vi "diffraction pattern v1.0.vi"() -> ()   [LabVIEW 2019]
panel:
  in  "Exit":bool
  in  "Run":bool
  out "Help":string="1. before run, set the paramaters on the left of the screen.\n2. flux (magnetic field) is in unit of flux quanta.\n3. Phaserange is in the unit of Pi, the CPR will be build up according to phase range of [-Phaserange/2,Phaserang/2], and such CPR will be  a periodic function with Phaserange as period. Enter integer number  of multiple times of 4 is preferred.\n4. Use the step setting tab to set resolution of the calculation, you can set how many points is used to define the width of the Josephson junction, how many points to represent the Phaserange\n5. Then you can choose which type of the CPR is used.\n6. Depending on the choose of the CPR, you may want to set the strength of the MBS, \"a\" parameter, the width of the gaussian function used, and the pattern of parity of MBS. Parity pattern has to have same number of elements for positive and negative range.\nEnter the parity 1 or -1 for positive and negative phase +-Pi, +-3Pi, +-5Pi etc.. in to the two arrays.\n7. You can use the index control to read the array elements, then enter the value, you can also delete an element of array by right click, the number of array elements is not limited.\n8. You can change the x,y range, zoom, create cursor etc. to help analyse the plot. Right click to save the data into excel.\n\nEnjoy!\nGuang Yue\n\n\n"
  in  "parity for negative phase":i32[](array[numeric])=[1, -1, -1, 1]
  in  "Strenth of MBS":dbl=0.5
  in  "parity for positive phase":i32[](array[numeric])=[1, -1, 1, 1]
  in  "Gaussian width":dbl=0.2
  in  "Tab Control":enum32{"Range", "Steps setting"}(tab)=enum."Steps setting"
  in  "flux start":dbl=-6.0
  in  "flux end":dbl=6.0
  in  "flux step":dbl=0.05
  in  "phaserange in Pi":i32=16
  in  "Geometry":i32=501
  in  "Phase steps":i32=501
  in  "CPR Type":T1(ring)=enum."Local MBS different parity"
  out "Total time s":dbl=20.42792349999945
  in  "stop loop":bool
  out "Diffraction pattern plot":cluster{cluster{dbl, "icn":dbl}[]}[](graph)=[{[{-6.0, "icn"=0.015201191288397739}, {-5.95, "icn"=0.01969262363818792}, {-5.9, "icn"=0.02816050403543407}, {-5.85, "icn"=0.03640577475812925}, {-5.8, "icn"=0.0442230884309362}, {-5.75, "icn"=0.05141409458211041}, {-5.7, "icn"=0.05779064505501809}, {-5.65, "icn"=0.06315912943628797}, {-5.6, "icn"=0.06721764065757277}, {-5.55, "icn"=0.06967553141250711}, {-5.5, "icn"=0.07013136060103732}, {-5.45, "icn"=0.06873370042025707}, {-5.4, "icn"=0.06529768198713366}, {-5.35, "icn"=0.06131135129764386}, {-5.3, "icn"=0.05712967537493866}, {-5.25, "icn"=0.05172563118780871}, {-5.2, "icn"=0.04512609278717199}, {-5.15, "icn"=0.03746288339324653}, {-5.1, "icn"=0.028906304270791668}, {-5.05, "icn"=0.019652598502870128}, {-5.0, "icn"=0.009919054928091782}, {-4.95, "icn"=0.01606737269953319}, {-4.9, "icn"=0.02621287150537696}, {-4.85, "icn"=0.036114718326525894}, {-4.8, "icn"=0.04552470847214177}, {-4.75, "icn"=0.05420143525490187}, {-4.7, "icn"=0.06191253761599668}, {-4.65, "icn"=0.06840325841911396}, {-4.6, "icn"=0.07337440089453802}, {-4.55, "icn"=0.07633960072265523}, {-4.5, "icn"=0.07694003757440993}, {-4.45, "icn"=0.07511288466626331}, {-4.4, "icn"=0.07094489106760657}, {-4.35, "icn"=0.06609689508373423}, {-4.3, "icn"=0.060931348029548554}, {-4.25, "icn"=0.05424909028223394}, {-4.2, "icn"=0.046059052595585265}, {-4.15, "icn"=0.03651979778138212}, {-4.1, "icn"=0.025834109202385443}, {-4.05, "icn"=0.014238092057178582}, {-4.0, "icn"=0.0019958503876323364}, {-3.9499999999999997, "icn"=0.010606220441872604}, {-3.9, "icn"=0.02326579038953691}, {-3.85, "icn"=0.03567147774513779}, {-3.8, "icn"=0.04751011276467433}, {-3.75, "icn"=0.05847437639350753}, {-3.6999999999999997, "icn"=0.06827384015050382}, {-3.65, "icn"=0.07669046186501231}, {-3.5999999999999996, "icn"=0.08435009902148928}, {-3.55, "icn"=0.09245040955594146}, {-3.5, "icn"=0.09818699818823985}, {-3.4499999999999997, "icn"=0.100890355120277}, {-3.4, "icn"=0.1004922625302631}, {-3.3499999999999996, "icn"=0.09706827829921433}, {-3.3, "icn"=0.09102426894947412}, {-3.25, "icn"=0.0827017030407996}, {-3.1999999999999997, "icn"=0.07233356294110323}, {-3.15, "icn"=0.06012975230451682}, {-3.0999999999999996, "icn"=0.046337743528162244}, {-3.05, "icn"=0.031250380479597245}, {-3.0, "icn"=0.015201191288398029}, {-2.9499999999999997, "icn"=0.02830046911314805}, {-2.9, "icn"=0.045606743446444754}, {-2.8499999999999996, "icn"=0.06271657669902271}, {-2.8, "icn"=0.07920905924934873}, {-2.75, "icn"=0.09466404490553904}, {-2.6999999999999997, "icn"=0.10868019873668189}, {-2.65, "icn"=0.12096184118712497}, {-2.5999999999999996, "icn"=0.13242531670888072}, {-2.55, "icn"=0.14449040955831893}, {-2.5, "icn"=0.15333287915372715}, {-2.4499999999999997, "icn"=0.15827148991751971}, {-2.4, "icn"=0.15853115847796279}, {-2.3499999999999996, "icn"=0.15489608459229445}, {-2.3, "icn"=0.1473321409279046}, {-2.25, "icn"=0.1364457543320676}, {-2.1999999999999997, "icn"=0.1224918472564987}, {-2.15, "icn"=0.10570069114472812}, {-2.0999999999999996, "icn"=0.0863674182534983}, {-2.05, "icn"=0.06485938540260895}, {-2.0, "icn"=0.04161187308992893}, {-1.9500000000000002, "icn"=0.06414199436705846}, {-1.8999999999999995, "icn"=0.09146312929875294}, {-1.8499999999999996, "icn"=0.11899756797085131}, {-1.7999999999999998, "icn"=0.1461262821875672}, {-1.75, "icn"=0.1722082272120952}, {-1.7000000000000002, "icn"=0.19658288396804854}, {-1.6499999999999995, "icn"=0.2184833976597425}, {-1.5999999999999996, "icn"=0.23659141533150718}, {-1.5499999999999998, "icn"=0.2498989153464729}, {-1.5, "icn"=0.2563220452314678}, {-1.4500000000000002, "icn"=0.2562842985268351}, {-1.3999999999999995, "icn"=0.24891519362535802}, {-1.3499999999999996, "icn"=0.2402432283340347}, {-1.2999999999999998, "icn"=0.22935682894260606}, {-1.25, "icn"=0.21279197567562266}, {-1.1999999999999993, "icn"=0.19021652655761598}, {-1.1499999999999995, "icn"=0.161624706006115}, {-1.0999999999999996, "icn"=0.12714683881730285}, {-1.0499999999999998, "icn"=0.0870252060665998}, {-1.0, "icn"=0.041611873089929}, {-0.9499999999999993, "icn"=0.09203583246104262}, {-0.8999999999999995, "icn"=0.15118411815627344}, {-0.8499999999999996, "icn"=0.21448578493954668}, {-0.7999999999999998, "icn"=0.28129040253853854}, {-0.75, "icn"=0.3508881885566983}, {-0.6999999999999993, "icn"=0.4224868106416624}, {-0.6499999999999995, "icn"=0.4948894711833411}, {-0.5999999999999996, "icn"=0.5661544315062148}, {-0.5499999999999998, "icn"=0.6323635438059886}, {-0.5, "icn"=0.6900329469436456}, {-0.4499999999999993, "icn"=0.7362703178024443}, {-0.39999999999999947, "icn"=0.7698525588790502}, {-0.34999999999999964, "icn"=0.810752483754053}, {-0.2999999999999998, "icn"=0.8578720391382381}, {-0.25, "icn"=0.8998638401870045}, {-0.1999999999999993, "icn"=0.9351626723633593}, {-0.14999999999999947, "icn"=0.9631769325077864}, {-0.09999999999999964, "icn"=0.9834888354480831}, {-0.04999999999999982, "icn"=0.9957976963002162}, {0.0, "icn"=0.9999210442038277}, {0.05000000000000071, "icn"=0.9957976963002159}, {0.10000000000000053, "icn"=0.9834888354480825}, {0.15000000000000036, "icn"=0.9631769325077865}, {0.20000000000000018, "icn"=0.9351626723633573}, {0.25, "icn"=0.8998638401870053}, {0.3000000000000007, "icn"=0.8578720391382365}, {0.35000000000000053, "icn"=0.8107524837540525}, {0.40000000000000036, "icn"=0.7698525588790497}, {0.4500000000000002, "icn"=0.7362703178024449}, {0.5, "icn"=0.6900329469436458}, {0.5500000000000007, "icn"=0.6323635438059875}, {0.6000000000000005, "icn"=0.5661544315062141}, {0.6500000000000004, "icn"=0.49488947118334015}, {0.7000000000000002, "icn"=0.42248681064166155}, {0.75, "icn"=0.35088818855669884}, {0.8000000000000007, "icn"=0.281290402538538}, {0.8500000000000005, "icn"=0.2144857849395455}, {0.9000000000000004, "icn"=0.1511841181562723}, {0.9500000000000002, "icn"=0.09203583246104151}, {1.0, "icn"=0.04161187308992913}, {1.0500000000000007, "icn"=0.08702520606660077}, {1.1000000000000005, "icn"=0.12714683881730346}, {1.1500000000000004, "icn"=0.16162470600611584}, {1.2000000000000002, "icn"=0.19021652655761667}, {1.25, "icn"=0.21279197567562247}, {1.3000000000000007, "icn"=0.22935682894260634}, {1.3500000000000005, "icn"=0.24024322833403497}, {1.4000000000000004, "icn"=0.24891519362535808}, {1.4500000000000002, "icn"=0.2562842985268354}, {1.5, "icn"=0.25632204523146773}, {1.5500000000000007, "icn"=0.24989891534647285}, {1.6000000000000005, "icn"=0.23659141533150693}, {1.6500000000000004, "icn"=0.21848339765974237}, {1.7000000000000002, "icn"=0.19658288396804882}, {1.75, "icn"=0.1722082272120953}, {1.8000000000000007, "icn"=0.14612628218756665}, {1.8500000000000005, "icn"=0.11899756797085088}, {1.9000000000000004, "icn"=0.09146312929875233}, {1.9500000000000002, "icn"=0.06414199436705838}, {2.0, "icn"=0.04161187308992881}, {2.0500000000000007, "icn"=0.06485938540260942}, {2.0999999999999996, "icn"=0.08636741825349839}, {2.1500000000000004, "icn"=0.10570069114472841}, {2.200000000000001, "icn"=0.12249184725649918}, {2.25, "icn"=0.13644575433206776}, {2.3000000000000007, "icn"=0.14733214092790461}, {2.3499999999999996, "icn"=0.15489608459229445}, {2.4000000000000004, "icn"=0.15853115847796276}, {2.450000000000001, "icn"=0.15827148991751952}, {2.5, "icn"=0.15333287915372706}, {2.5500000000000007, "icn"=0.14449040955831877}, {2.5999999999999996, "icn"=0.13242531670888066}, {2.6500000000000004, "icn"=0.12096184118712507}, {2.700000000000001, "icn"=0.10868019873668154}, {2.75, "icn"=0.09466404490553902}, {2.8000000000000007, "icn"=0.0792090592493484}, {2.8499999999999996, "icn"=0.06271657669902268}, {2.9000000000000004, "icn"=0.04560674344644471}, {2.950000000000001, "icn"=0.02830046911314761}, {3.0, "icn"=0.015201191288398011}, {3.0500000000000007, "icn"=0.03125038047959755}, {3.0999999999999996, "icn"=0.046337743528162154}, {3.1500000000000004, "icn"=0.06012975230451701}, {3.200000000000001, "icn"=0.07233356294110352}, {3.25, "icn"=0.08270170304079963}, {3.3000000000000007, "icn"=0.09102426894947409}, {3.3499999999999996, "icn"=0.09706827829921418}, {3.4000000000000004, "icn"=0.10049226253026292}, {3.450000000000001, "icn"=0.10089035512027685}, {3.5, "icn"=0.09818699818823978}, {3.5500000000000007, "icn"=0.09245040955594122}, {3.6000000000000014, "icn"=0.08435009902148892}, {3.6500000000000004, "icn"=0.07669046186501216}, {3.700000000000001, "icn"=0.06827384015050363}, {3.75, "icn"=0.058474376393507374}, {3.8000000000000007, "icn"=0.04751011276467419}, {3.8500000000000014, "icn"=0.035671477745137556}, {3.9000000000000004, "icn"=0.023265790389536557}, {3.950000000000001, "icn"=0.010606220441872458}, {4.0, "icn"=0.001995850387632321}, {4.050000000000001, "icn"=0.014238092057178757}, {4.100000000000001, "icn"=0.025834109202385887}, {4.15, "icn"=0.03651979778138197}, {4.200000000000001, "icn"=0.046059052595585515}, {4.25, "icn"=0.05424909028223394}, {4.300000000000001, "icn"=0.060931348029548776}, {4.350000000000001, "icn"=0.06609689508373423}, {4.4, "icn"=0.07094489106760664}, {4.450000000000001, "icn"=0.07511288466626348}, {4.5, "icn"=0.07694003757440998}, {4.550000000000001, "icn"=0.0763396007226551}, {4.600000000000001, "icn"=0.07337440089453792}, {4.65, "icn"=0.06840325841911381}, {4.700000000000001, "icn"=0.06191253761599665}, {4.75, "icn"=0.05420143525490175}, {4.800000000000001, "icn"=0.04552470847214158}, {4.850000000000001, "icn"=0.036114718326525366}, {4.9, "icn"=0.026212871505376868}, {4.950000000000001, "icn"=0.01606737269953315}, {5.0, "icn"=0.009919054928091796}, {5.050000000000001, "icn"=0.019652598502870263}, {5.100000000000001, "icn"=0.028906304270791987}, {5.15, "icn"=0.03746288339324643}, {5.200000000000001, "icn"=0.045126092787172174}, {5.25, "icn"=0.05172563118780869}, {5.300000000000001, "icn"=0.057129675374938675}, {5.350000000000001, "icn"=0.06131135129764395}, {5.4, "icn"=0.06529768198713373}, {5.450000000000001, "icn"=0.06873370042025718}, {5.5, "icn"=0.07013136060103738}, {5.550000000000001, "icn"=0.0696755314125071}, {5.600000000000001, "icn"=0.06721764065757257}, {5.65, "icn"=0.06315912943628808}, {5.700000000000001, "icn"=0.05779064505501793}, {5.75, "icn"=0.051414094582110305}, {5.800000000000001, "icn"=0.04422308843093613}, {5.850000000000001, "icn"=0.03640577475812903}, {5.9, "icn"=0.028160504035433992}, {5.950000000000001, "icn"=0.019692623638187533}, {6.0, "icn"=0.015201191288397769}]}, {[{-6.0, "icn"=-0.015201191288398015}, {-5.95, "icn"=-0.019692623638187804}, {-5.9, "icn"=-0.02816050403543406}, {-5.85, "icn"=-0.036405774758129165}, {-5.8, "icn"=-0.04422308843093618}, {-5.75, "icn"=-0.05141409458211045}, {-5.7, "icn"=-0.05779064505501804}, {-5.65, "icn"=-0.06315912943628808}, {-5.6, "icn"=-0.06721764065757263}, {-5.55, "icn"=-0.06967553141250715}, {-5.5, "icn"=-0.0701313606010374}, {-5.45, "icn"=-0.06873370042025713}, {-5.4, "icn"=-0.06529768198713366}, {-5.35, "icn"=-0.061311351297643965}, {-5.3, "icn"=-0.05712967537493852}, {-5.25, "icn"=-0.05172563118780883}, {-5.2, "icn"=-0.04512609278717185}, {-5.15, "icn"=-0.037462883393246306}, {-5.1, "icn"=-0.02890630427079172}, {-5.05, "icn"=-0.01965259850287017}, {-5.0, "icn"=-0.009919054928091801}, {-4.95, "icn"=-0.01606737269953315}, {-4.9, "icn"=-0.026212871505377}, {-4.85, "icn"=-0.036114718326525866}, {-4.8, "icn"=-0.045524708472141566}, {-4.75, "icn"=-0.05420143525490171}, {-4.7, "icn"=-0.061912537615996494}, {-4.65, "icn"=-0.06840325841911382}, {-4.6, "icn"=-0.07337440089453802}, {-4.55, "icn"=-0.07633960072265512}, {-4.5, "icn"=-0.07694003757441016}, {-4.45, "icn"=-0.07511288466626329}, {-4.4, "icn"=-0.07094489106760672}, {-4.35, "icn"=-0.06609689508373419}, {-4.3, "icn"=-0.060931348029548596}, {-4.25, "icn"=-0.05424909028223398}, {-4.2, "icn"=-0.04605905259558536}, {-4.15, "icn"=-0.03651979778138199}, {-4.1, "icn"=-0.025834109202385432}, {-4.05, "icn"=-0.014238092057178612}, {-4.0, "icn"=-0.0019958503876324305}, {-3.9499999999999997, "icn"=-0.010606220441872783}, {-3.9, "icn"=-0.02326579038953663}, {-3.85, "icn"=-0.03567147774513782}, {-3.8, "icn"=-0.047510112764674456}, {-3.75, "icn"=-0.05847437639350741}, {-3.6999999999999997, "icn"=-0.06827384015050389}, {-3.65, "icn"=-0.07669046186501216}, {-3.5999999999999996, "icn"=-0.08435009902148922}, {-3.55, "icn"=-0.09245040955594135}, {-3.5, "icn"=-0.09818699818823987}, {-3.4499999999999997, "icn"=-0.10089035512027698}, {-3.4, "icn"=-0.10049226253026303}, {-3.3499999999999996, "icn"=-0.09706827829921416}, {-3.3, "icn"=-0.09102426894947405}, {-3.25, "icn"=-0.08270170304079953}, {-3.1999999999999997, "icn"=-0.07233356294110314}, {-3.15, "icn"=-0.06012975230451686}, {-3.0999999999999996, "icn"=-0.04633774352816224}, {-3.05, "icn"=-0.03125038047959716}, {-3.0, "icn"=-0.015201191288398325}, {-2.9499999999999997, "icn"=-0.028300469113147916}, {-2.9, "icn"=-0.04560674344644478}, {-2.8499999999999996, "icn"=-0.06271657669902267}, {-2.8, "icn"=-0.07920905924934862}, {-2.75, "icn"=-0.09466404490553891}, {-2.6999999999999997, "icn"=-0.10868019873668189}, {-2.65, "icn"=-0.120961841187125}, {-2.5999999999999996, "icn"=-0.13242531670888058}, {-2.55, "icn"=-0.144490409558319}, {-2.5, "icn"=-0.1533328791537271}, {-2.4499999999999997, "icn"=-0.15827148991751958}, {-2.4, "icn"=-0.15853115847796273}, {-2.3499999999999996, "icn"=-0.1548960845922946}, {-2.3, "icn"=-0.1473321409279045}, {-2.25, "icn"=-0.13644575433206824}, {-2.1999999999999997, "icn"=-0.12249184725649886}, {-2.15, "icn"=-0.10570069114472823}, {-2.0999999999999996, "icn"=-0.08636741825349832}, {-2.05, "icn"=-0.06485938540260898}, {-2.0, "icn"=-0.04161187308992876}, {-1.9500000000000002, "icn"=-0.0641419943670583}, {-1.8999999999999995, "icn"=-0.09146312929875272}, {-1.8499999999999996, "icn"=-0.11899756797085136}, {-1.7999999999999998, "icn"=-0.1461262821875672}, {-1.75, "icn"=-0.17220822721209544}, {-1.7000000000000002, "icn"=-0.1965828839680486}, {-1.6499999999999995, "icn"=-0.21848339765974256}, {-1.5999999999999996, "icn"=-0.23659141533150688}, {-1.5499999999999998, "icn"=-0.24989891534647296}, {-1.5, "icn"=-0.25632204523146807}, {-1.4500000000000002, "icn"=-0.25628429852683515}, {-1.3999999999999995, "icn"=-0.24891519362535786}, {-1.3499999999999996, "icn"=-0.24024322833403494}, {-1.2999999999999998, "icn"=-0.22935682894260628}, {-1.25, "icn"=-0.21279197567562225}, {-1.1999999999999993, "icn"=-0.19021652655761598}, {-1.1499999999999995, "icn"=-0.16162470600611525}, {-1.0999999999999996, "icn"=-0.12714683881730265}, {-1.0499999999999998, "icn"=-0.08702520606659991}, {-1.0, "icn"=-0.04161187308992906}, {-0.9499999999999993, "icn"=-0.09203583246104254}, {-0.8999999999999995, "icn"=-0.15118411815627344}, {-0.8499999999999996, "icn"=-0.21448578493954695}, {-0.7999999999999998, "icn"=-0.281290402538539}, {-0.75, "icn"=-0.3508881885566993}, {-0.6999999999999993, "icn"=-0.4224868106416633}, {-0.6499999999999995, "icn"=-0.49488947118334164}, {-0.5999999999999996, "icn"=-0.5661544315062156}, {-0.5499999999999998, "icn"=-0.6323635438059881}, {-0.5, "icn"=-0.6900329469436459}, {-0.4499999999999993, "icn"=-0.736270317802446}, {-0.39999999999999947, "icn"=-0.76985255887905}, {-0.34999999999999964, "icn"=-0.8107524837540534}, {-0.2999999999999998, "icn"=-0.8578720391382376}, {-0.25, "icn"=-0.899863840187005}, {-0.1999999999999993, "icn"=-0.9351626723633584}, {-0.14999999999999947, "icn"=-0.963176932507787}, {-0.09999999999999964, "icn"=-0.9834888354480829}, {-0.04999999999999982, "icn"=-0.9957976963002159}, {0.0, "icn"=-0.9999210442038277}, {0.05000000000000071, "icn"=-0.9957976963002162}, {0.10000000000000053, "icn"=-0.9834888354480825}, {0.15000000000000036, "icn"=-0.9631769325077862}, {0.20000000000000018, "icn"=-0.9351626723633589}, {0.25, "icn"=-0.8998638401870043}, {0.3000000000000007, "icn"=-0.8578720391382374}, {0.35000000000000053, "icn"=-0.810752483754052}, {0.40000000000000036, "icn"=-0.7698525588790498}, {0.4500000000000002, "icn"=-0.7362703178024443}, {0.5, "icn"=-0.6900329469436454}, {0.5500000000000007, "icn"=-0.6323635438059875}, {0.6000000000000005, "icn"=-0.5661544315062141}, {0.6500000000000004, "icn"=-0.4948894711833398}, {0.7000000000000002, "icn"=-0.4224868106416615}, {0.75, "icn"=-0.3508881885566994}, {0.8000000000000007, "icn"=-0.2812904025385381}, {0.8500000000000005, "icn"=-0.21448578493954548}, {0.9000000000000004, "icn"=-0.1511841181562722}, {0.9500000000000002, "icn"=-0.09203583246104138}, {1.0, "icn"=-0.04161187308992905}, {1.0500000000000007, "icn"=-0.0870252060666006}, {1.1000000000000005, "icn"=-0.1271468388173035}, {1.1500000000000004, "icn"=-0.1616247060061158}, {1.2000000000000002, "icn"=-0.1902165265576164}, {1.25, "icn"=-0.21279197567562255}, {1.3000000000000007, "icn"=-0.22935682894260648}, {1.3500000000000005, "icn"=-0.2402432283340353}, {1.4000000000000004, "icn"=-0.24891519362535805}, {1.4500000000000002, "icn"=-0.25628429852683515}, {1.5, "icn"=-0.2563220452314681}, {1.5500000000000007, "icn"=-0.24989891534647274}, {1.6000000000000005, "icn"=-0.23659141533150685}, {1.6500000000000004, "icn"=-0.21848339765974215}, {1.7000000000000002, "icn"=-0.1965828839680484}, {1.75, "icn"=-0.17220822721209533}, {1.8000000000000007, "icn"=-0.1461262821875665}, {1.8500000000000005, "icn"=-0.11899756797085094}, {1.9000000000000004, "icn"=-0.0914631292987523}, {1.9500000000000002, "icn"=-0.06414199436705846}, {2.0, "icn"=-0.04161187308992888}, {2.0500000000000007, "icn"=-0.06485938540260934}, {2.0999999999999996, "icn"=-0.08636741825349825}, {2.1500000000000004, "icn"=-0.10570069114472827}, {2.200000000000001, "icn"=-0.12249184725649909}, {2.25, "icn"=-0.1364457543320682}, {2.3000000000000007, "icn"=-0.1473321409279047}, {2.3499999999999996, "icn"=-0.15489608459229462}, {2.4000000000000004, "icn"=-0.1585311584779625}, {2.450000000000001, "icn"=-0.1582714899175197}, {2.5, "icn"=-0.1533328791537272}, {2.5500000000000007, "icn"=-0.14449040955831854}, {2.5999999999999996, "icn"=-0.13242531670888058}, {2.6500000000000004, "icn"=-0.12096184118712493}, {2.700000000000001, "icn"=-0.10868019873668144}, {2.75, "icn"=-0.09466404490553901}, {2.8000000000000007, "icn"=-0.0792090592493484}, {2.8499999999999996, "icn"=-0.06271657669902266}, {2.9000000000000004, "icn"=-0.0456067434464448}, {2.950000000000001, "icn"=-0.028300469113147594}, {3.0, "icn"=-0.015201191288398386}, {3.0500000000000007, "icn"=-0.03125038047959767}, {3.0999999999999996, "icn"=-0.046337743528162244}, {3.1500000000000004, "icn"=-0.060129752304517066}, {3.200000000000001, "icn"=-0.07233356294110345}, {3.25, "icn"=-0.08270170304079963}, {3.3000000000000007, "icn"=-0.09102426894947413}, {3.3499999999999996, "icn"=-0.09706827829921426}, {3.4000000000000004, "icn"=-0.10049226253026296}, {3.450000000000001, "icn"=-0.10089035512027694}, {3.5, "icn"=-0.09818699818823999}, {3.5500000000000007, "icn"=-0.09245040955594123}, {3.6000000000000014, "icn"=-0.08435009902148902}, {3.6500000000000004, "icn"=-0.07669046186501215}, {3.700000000000001, "icn"=-0.06827384015050374}, {3.75, "icn"=-0.05847437639350735}, {3.8000000000000007, "icn"=-0.047510112764674275}, {3.8500000000000014, "icn"=-0.03567147774513749}, {3.9000000000000004, "icn"=-0.023265790389536665}, {3.950000000000001, "icn"=-0.010606220441872365}, {4.0, "icn"=-0.00199585038763244}, {4.050000000000001, "icn"=-0.014238092057178922}, {4.100000000000001, "icn"=-0.025834109202385897}, {4.15, "icn"=-0.036519797781382146}, {4.200000000000001, "icn"=-0.04605905259558554}, {4.25, "icn"=-0.05424909028223402}, {4.300000000000001, "icn"=-0.06093134802954878}, {4.350000000000001, "icn"=-0.06609689508373429}, {4.4, "icn"=-0.0709448910676066}, {4.450000000000001, "icn"=-0.07511288466626342}, {4.5, "icn"=-0.07694003757441015}, {4.550000000000001, "icn"=-0.07633960072265515}, {4.600000000000001, "icn"=-0.07337440089453791}, {4.65, "icn"=-0.06840325841911385}, {4.700000000000001, "icn"=-0.06191253761599663}, {4.75, "icn"=-0.0542014352549018}, {4.800000000000001, "icn"=-0.04552470847214147}, {4.850000000000001, "icn"=-0.036114718326525484}, {4.9, "icn"=-0.026212871505377}, {4.950000000000001, "icn"=-0.01606737269953297}, {5.0, "icn"=-0.00991905492809179}, {5.050000000000001, "icn"=-0.019652598502870305}, {5.100000000000001, "icn"=-0.028906304270792004}, {5.15, "icn"=-0.037462883393246375}, {5.200000000000001, "icn"=-0.04512609278717223}, {5.25, "icn"=-0.05172563118780885}, {5.300000000000001, "icn"=-0.057129675374938585}, {5.350000000000001, "icn"=-0.06131135129764406}, {5.4, "icn"=-0.06529768198713364}, {5.450000000000001, "icn"=-0.06873370042025705}, {5.5, "icn"=-0.0701313606010373}, {5.550000000000001, "icn"=-0.06967553141250703}, {5.600000000000001, "icn"=-0.06721764065757253}, {5.65, "icn"=-0.06315912943628801}, {5.700000000000001, "icn"=-0.05779064505501793}, {5.75, "icn"=-0.05141409458211044}, {5.800000000000001, "icn"=-0.04422308843093607}, {5.850000000000001, "icn"=-0.03640577475812899}, {5.9, "icn"=-0.02816050403543421}, {5.950000000000001, "icn"=-0.019692623638187787}, {6.0, "icn"=-0.015201191288397961}]}]
  out "Ic negative":dbl=-0.015201191288397961
  out "Ic positive":dbl=0.015201191288397769
  out "error out":errorcluster
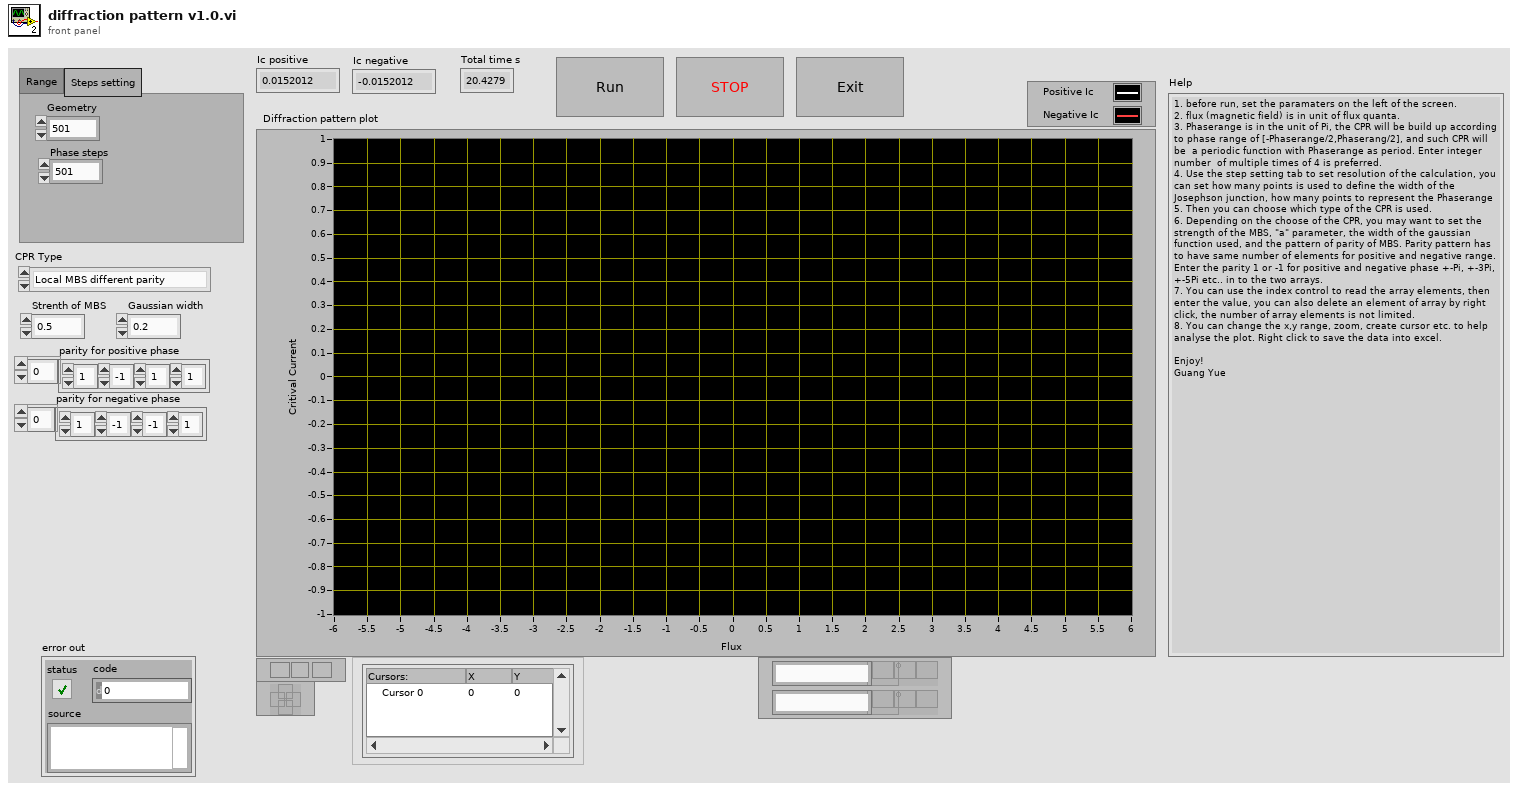
[diagram p1: front panel]
types:
  T1 = enum16{"Regular Josephson effect", "Non-local MBS", "Local MBS same parity", "Local MBS different parity"}
  T2 = enum32{"invalid app kind", "Development System", "Run Time System", "Student Edition", "Embedded LabVIEW", "Evaluation", "Custom"}
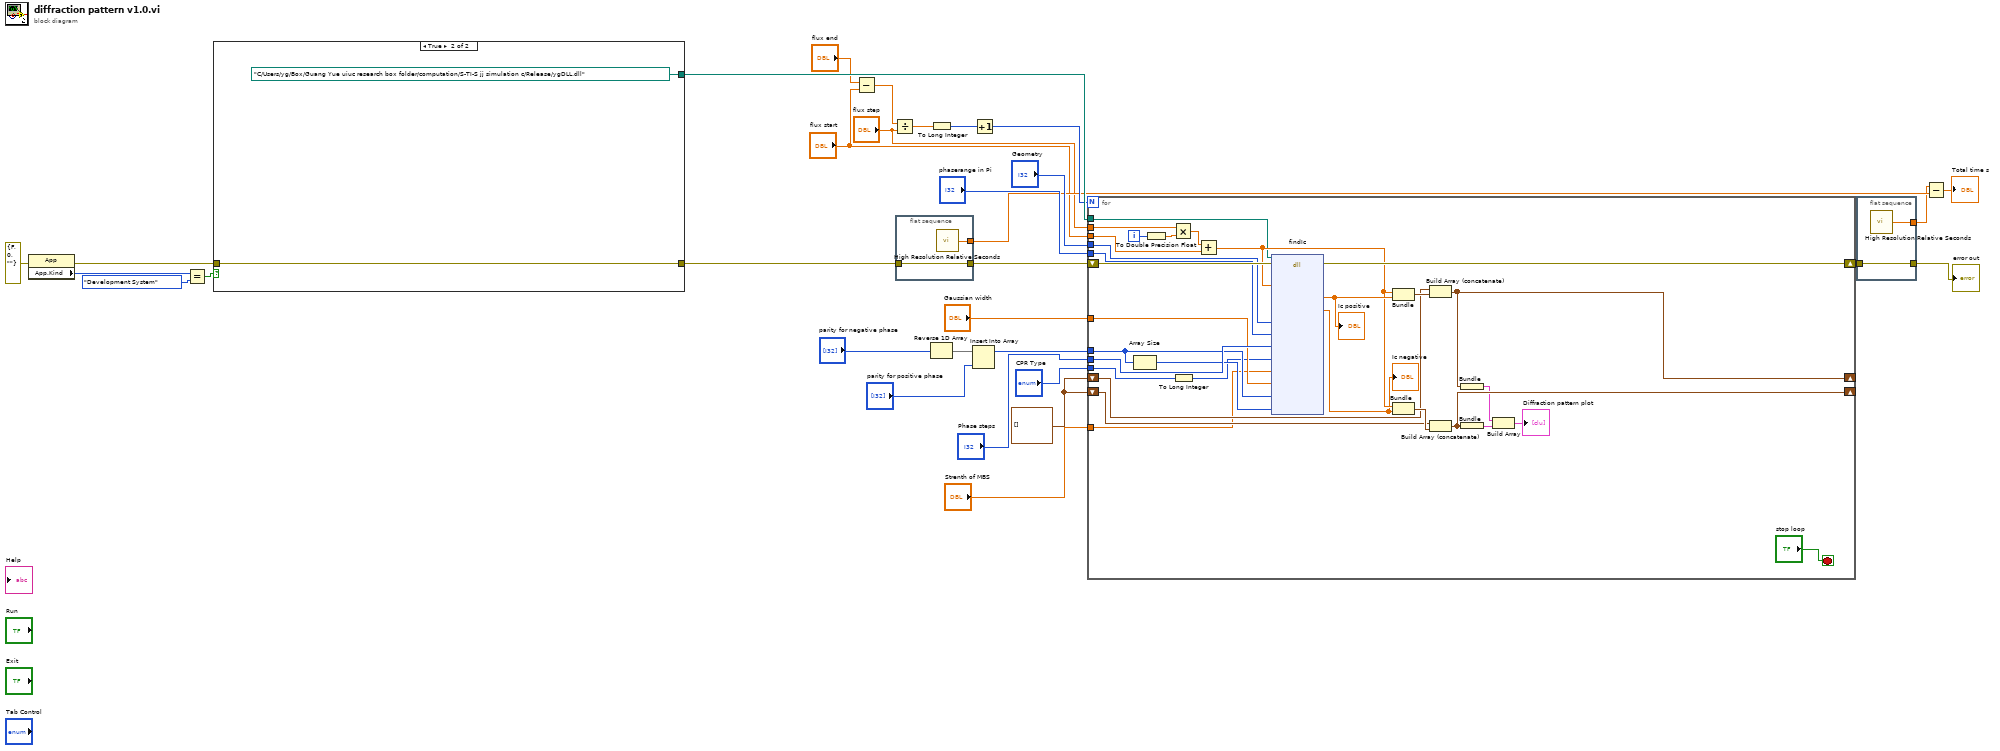
[diagram p0: block diagram]
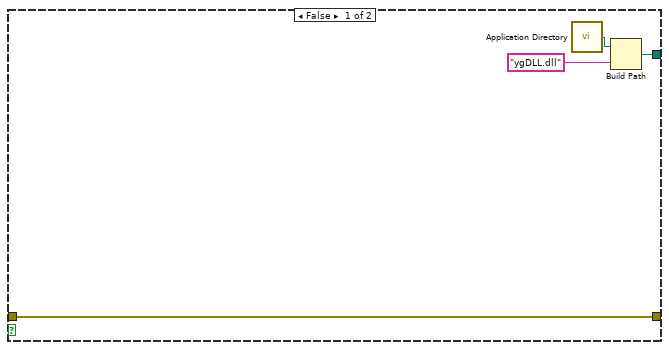
[diagram p2: hidden frame]
diagram:
  w2 = cluster{dbl, "inp":dbl}[] []
  n1 = property class="App"(error in=errorcluster {"status"=FALSE, "code"=0, "source"=""} ("error out")) -> (error out=w27:errorcluster, "App.Kind"=w30:T2)  [unwired: 1 in, 1 out]
  n2 = Equal?(x=w30, y=T2."Development System" ("Application:Kind")) -> (x = y?=w28:bool)
  n3 = case shown="True" w28 {
    tunnel: [w33 path "C:/Users/yg/Box/Guang Yue uiuc research box folder/computation/S-TI-S jj simulation c/Release/ygDLL.dll"] -> w25
    tunnel: w27 -> [w32 w36]
    tunnel: [w32 w36] -> w26
    frame False {
      n4 = call <vilib>:"Application Directory.vi"() -> ("Application Directory"=w35:path)
      n5 = Build Path(base path=w35, name or relative path="ygDLL.dll") -> (appended path=w33:path)
    }
    frame True {
    }
  }
  n6 = Subtract(x="flux end", y="flux start") -> (x-y=w4:dbl)
  n7 = Divide(x=w4, y="flux step") -> (x/y=w5:dbl)
  n8 = flat-sequence {
    tunnel: w26 -> [w39]
    tunnel: [w39] -> w9
    tunnel: [w38] -> w12
    frame #0 {
      n9 = call <vilib>:"High Resolution Relative Seconds.vi"() -> ("relative seconds"=w38:dbl)
    }
  }
  n10 = To Long Integer(number=w5) -> (32bit integer=w6:i32)
  n11 = Reverse 1D Array(array="parity for negative phase") -> (reversed array=w21:i32[])
  n12 = Insert Into Array(array=w21, new element="parity for positive phase") -> (w23:i32[])  [unwired: 1 in]
  n13 = Increment(x=w6) -> (x+1=w19:i32)
  n14 = for {
    N: w19 -> [_]
    shift-right: [w69] -> w10
    shift-left: w9 -> [w68]
    tunnel: "flux step" -> [w66]
    tunnel: "flux start" -> [w63]
    shift-right: [w54] -> _
    shift-left: w2 -> [w56]
    shift-right: [w53] -> _
    shift-left: w2 -> [w55]
    tunnel: w25 -> [w49]
    tunnel: "Geometry" -> [w48]
    tunnel: "phaserange in Pi" -> [w47]
    tunnel: "Phase steps" -> [w46]
    tunnel: "CPR Type" -> [w45]
    tunnel: "Gaussian width" -> [w44]
    tunnel: w23 -> [w43]
    tunnel: "Strenth of MBS" -> [w41]
    i -> [w67]
    stop <- "stop loop" stop-if-true
    n15 = Array Size(array=w43) -> (size(s)=w42:i32)
    n16 = To Double Precision Float(number=w67) -> (double precision float=w65:dbl)
    n17 = Multiply(x=w66, y=w65) -> (x*y=w64:dbl)
    n18 = To Long Integer(number=w45) -> (32bit integer=w40:i32)
    n19 = Add(x=w64, y=w63) -> (x+y=w60:dbl)
    n20 = dll-call lib="C:/Users/yg/Box/Guang Yue uiuc research box folder/computation/S-TI-S jj simulation c/Release/ygDLL.dll" fn="findIc"(path in=w49, error in=w68, "flux"=w60, "nw"=w48, "phaserange"=w47, "nphase"=w46, "cpr"=w40, "a"=w41, "gw"=w44, "parity"=w43, "parity_l"=w42) -> (error out=w69:errorcluster, "inp"=w61:dbl, "icn"=w59:dbl)  [unwired: 13 in, 1 out]
    "Ic positive" <- w61
    "Ic negative" <- w59
    n21 = Bundle(w60, "inp"=w61) -> (w58:cluster{dbl, "inp":dbl})  [unwired: 1 in]
    n22 = Bundle(w60, "icn"=w59) -> (w57:cluster{dbl, "icn":dbl})  [unwired: 1 in]
    n23 = Build Array (concatenate)(w56, w58) -> (w54:cluster{dbl, "inp":dbl}[])
    n24 = Build Array (concatenate)(w55, w57) -> (w53:cluster{dbl, "icn":dbl}[])
    n25 = Bundle(w54) -> (w52:cluster{cluster{dbl, "inp":dbl}[]})  [unwired: 1 in]
    n26 = Bundle(w53) -> (w51:cluster{cluster{dbl, "icn":dbl}[]})  [unwired: 1 in]
    n27 = Build Array(w52, w51) -> (→"Diffraction pattern plot":cluster{cluster{dbl, "icn":dbl}[]}[])
  }
  n28 = flat-sequence {
    tunnel: w10 -> [w71]
    tunnel: [w71] -> w1
    tunnel: [w70] -> w11
    frame #0 {
      n29 = call <vilib>:"High Resolution Relative Seconds.vi"() -> ("relative seconds"=w70:dbl)
    }
  }
  n30 = Subtract(x=w11, y=w12) -> (x-y=→"Total time s":dbl)
  "error out" <- w1
